vi "Day 2.1 - ..vi"(11 "input":string[](array[string])) -> (3 "ouptut part 1":u64)   [LabVIEW 2021]
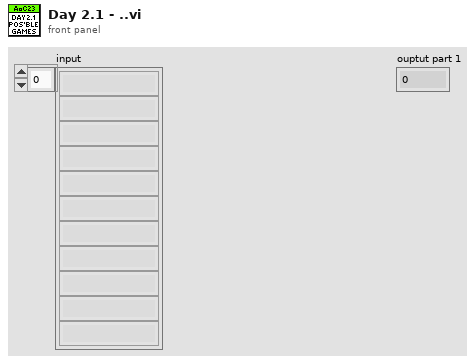
[diagram p1: front panel]
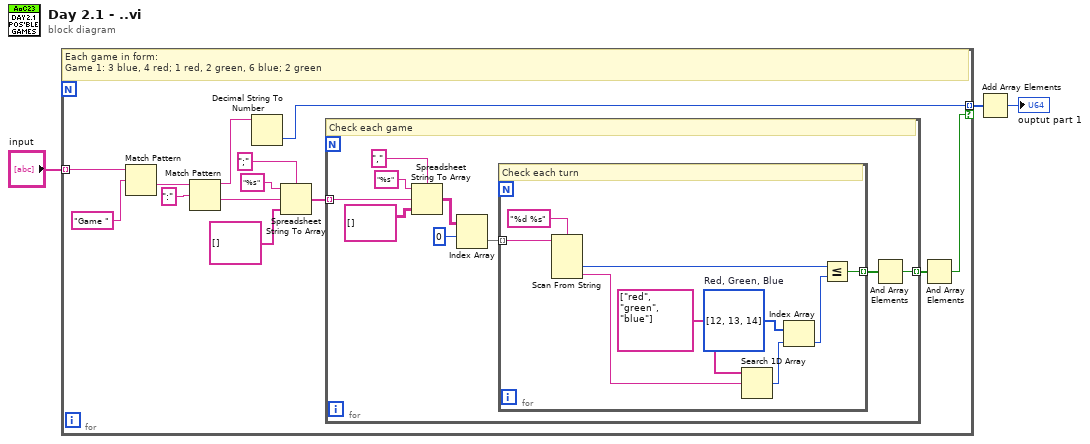
[diagram p0: block diagram]
diagram:
  n1 = for {
    tunnel: "input" -> [w13] mode=indexing
    tunnel: [w8] -> w2 mode=indexing if=w4
    # "Each game in form:\nGame 1: 3 blue, 4 red; 1 red, 2 green, 6 blue; 2 green"
    n2 = Match Pattern(string=w13, regular expression="Game ") -> (after substring=w11:string)  [unwired: 1 in, 3 out]
    n3 = Match Pattern(string=w11, regular expression=":") -> (before substring=w9:string, after substring=w7:string)  [unwired: 1 in, 2 out]
    n4 = Decimal String To Number(string=w9) -> (number=w8:i32)  [unwired: 2 in, 1 out]
    n5 = Spreadsheet String To Array(delimiter (Tab)=";", format string="%s", spreadsheet string=w7, array type (2D Dbl)=string[] []) -> (array=w6:string[])
    n6 = for {
      tunnel: w6 -> [w25] mode=indexing
      tunnel: [w17] -> w5 mode=indexing
      # "Check each game"
      n7 = Spreadsheet String To Array(delimiter (Tab)=",", format string="%s", spreadsheet string=w25, array type (2D Dbl)=string[][] []) -> (array=w21:string[][])
      n8 = Index Array(array=w21, index (row)=0) -> (element=w19:string[])  [unwired: 1 in]
      n9 = for {
        tunnel: w19 -> [w33] mode=indexing
        tunnel: [w27] -> w18 mode=indexing
        w31 = i32[] [12, 13, 14]  # Red, Green, Blue
        # "Check each turn"
        n10 = Scan From String(format string="%d %s", input string=w33) -> (output 1=w29:i32, output 2=w32:string)  [unwired: 4 in, 3 out]
        n11 = Search 1D Array(1D array=string[] ["red", "green", "blue"], element=w32) -> (index of element=w30:i32)  [unwired: 1 in]
        n12 = Index Array(array=w31, index=w30) -> (element=w28:i32)
        n13 = Less Or Equal?(x=w29, y=w28) -> (x <= y?=w27:bool)
      }
      n14 = And Array Elements(Boolean array=w18) -> (logical AND=w17:bool)
    }
    n15 = And Array Elements(Boolean array=w5) -> (logical AND=w4:bool)
  }
  n16 = Add Array Elements(numeric array=w2) -> (sum=→"ouptut part 1":i32)
